vi "Flatten Value.vi"(8 "Error In":errorcluster, 11 "2D Flt In":refnum<class "2D Flt.lvclass">) -> (0 "Error Out":errorcluster, 1 "Value":string, 3 "2D Flt Out":refnum<class "2D Flt.lvclass">)   [LabVIEW 2017, in "Tree API.lvlib" / "2D Flt.lvclass"]
doc: "Dynamic dispatch interface for flattening Tree Data classes to string."
uses:
  2D Flt.lvclass
  Tree Manager/Tree.lvclass
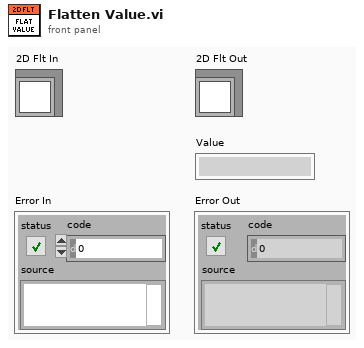
[diagram p1: front panel]
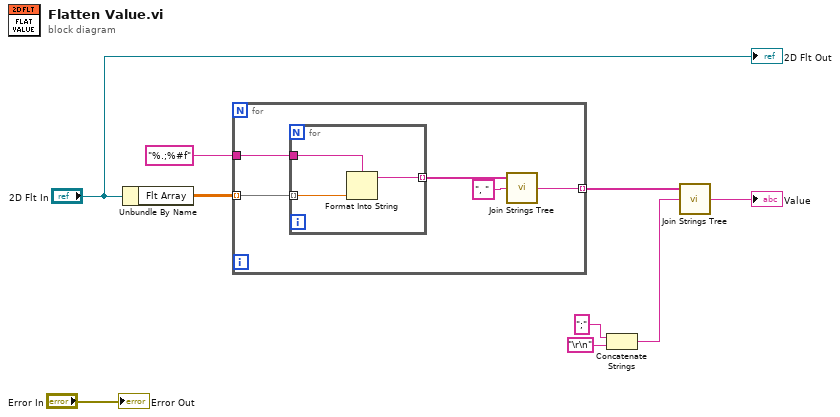
[diagram p0: block diagram]
diagram:
  n1 = Unbundle By Name("2D Flt In") -> ("Flt Array"=w8:dbl[][])
  n2 = for {
    tunnel: w8 -> [w14] mode=indexing
    tunnel: [w11] -> w9 mode=indexing
    tunnel: "%.;%#f" ("initial string") -> [w10]
    n3 = for {
      tunnel: w14 -> [w17] mode=indexing
      tunnel: [w16] -> w13 mode=indexing
      tunnel: w10 -> [w15]
      n4 = Format Into String(format string=w15, w17) -> (resulting string=w16:string)  [unwired: 2 in, 1 out]
    }
    n5 = call "Join Strings Tree.vi"("Separator (,)"=", ", "Strings In"=w13) -> ("String"=w11:string)  [unwired: 1 in]
  }
  n6 = Concatenate Strings(";" ("Separator (,)"), "\r\n") -> (w2:string)
  n7 = call "Join Strings Tree.vi"("Separator (,)"=w2, "Strings In"=w9) -> ("String"=→"Value":string)  [unwired: 1 in]
  "2D Flt Out" <- "2D Flt In"
  "Error Out" <- "Error In"
